vi "Select_baudios_SerialRS232.vi"(1 "Baudios":T1(ring)) -> (0 "baud rate (9600)":u32)   [LabVIEW 2019]
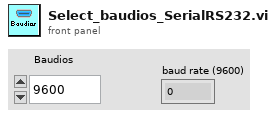
[diagram p1: front panel]
types:
  T1 = enum16{"9600", "14400", "19200", "38400", "56000", "57600", "115200"}
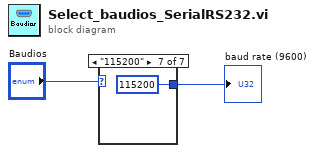
[diagram p0: block diagram]
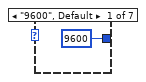
[diagram p2: hidden frame]
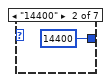
[diagram p3: hidden frame]
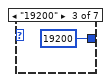
[diagram p4: hidden frame]
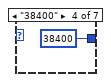
[diagram p5: hidden frame]
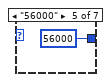
[diagram p6: hidden frame]
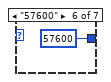
[diagram p7: hidden frame]
diagram:
  n1 = case shown="\"115200\"" "Baudios" {
    tunnel: [u32 9600 ("baud rate (9600)") u32 14400 ("baud rate (9600)") u32 19200 ("baud rate (9600)") u32 38400 ("baud rate (9600)") u32 56000 ("baud rate (9600)") u32 57600 ("baud rate (9600)") u32 115200 ("baud rate (9600)")] -> w1
    frame "9600", Default {
    }
    frame "14400" {
    }
    frame "19200" {
    }
    frame "38400" {
    }
    frame "56000" {
    }
    frame "57600" {
    }
    frame "115200" {
    }
  }
  "baud rate (9600)" <- w1
